vi "WriteSingleJoint.vi"(0 "Angle Name":T1(ring), 1 "node":string, 2 "Angle (degrees)":dbl, 3 "error in":errorcluster, 4 "Mode":T2=1 items=["Position"=1, "Velocity"=2, "Effort"=3]) -> (6 "error out":errorcluster)   [LabVIEW 2010]
uses:
  ROS/Code/SubVIs/_ROSDirection.ctl
  ROS/Code/Console/Servers/ServerSubs/TopicDef.ctl
  ROS/MessageBuilding/std_msgs/subs/i32Scalar.vi
  ROS/MessageBuilding/std_msgs/subs/float64Array.vi
  ROS/MessageBuilding/std_msgs/subs/stringArray.vi
  ROS/Code/SubVIs/JointMode.ctl
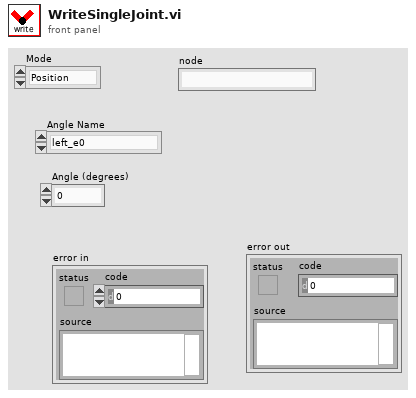
[diagram p1: front panel]
types:
  T1 = enum16{"left_e0", "left_e1", "left_s0", "left_s1", "left_w0", "left_w1", "left_w2", "right_e0", "right_e1", "right_s0", "right_s1", "right_w0", "right_w1", "right_w2"}
  T2 = typedef "JointMode.ctl" = u8
  T3 = typedef "TopicDef.ctl" = cluster{"Topic":string, "Type":string, "Action":T4, "Update (ms)":u16, "write queue":u16}
  T4 = typedef "_ROSDirection.ctl" = enum16{"Node", "Publisher", "Subscriber", "Service Client"}
  T5 = typedef "_ROSControl.ctl" = cluster{"topic port":u16, "Node":string, "topic":string, "type":string, "node port":u32, "error ":errorcluster, "Direction":T4, "APIs":string[], "Update (ms)":u16, "write queue":u16}
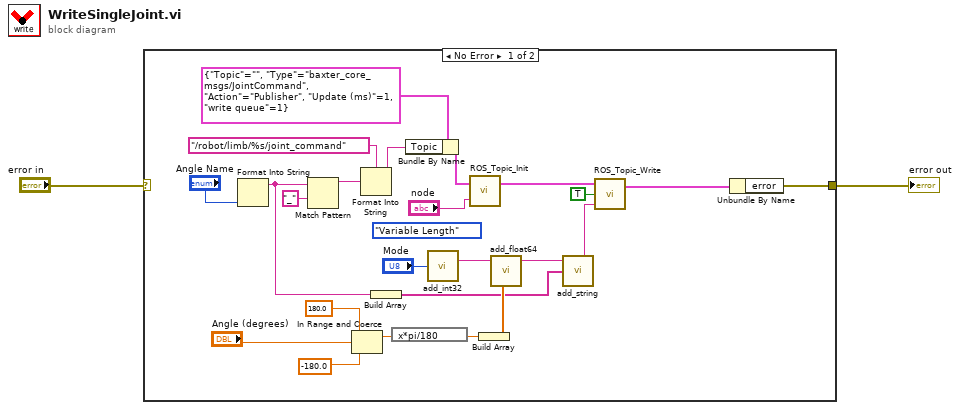
[diagram p0: block diagram]
diagram:
  n1 = case shown="No Error" "error in" {
    selector: "error in" -> [_ w27]
    tunnel: [w26 w27] -> w2
    frame No Error {
      (unwired) enum16{"Fixed Length", "Variable Length"}."Variable Length" ("Array Type")
      n2 = Format Into String("Angle Name") -> (resulting string=w6:string)  [unwired: 3 in, 1 out]
      n3 = Match Pattern(string=w6, regular expression="_") -> (before substring=w11:string)  [unwired: 1 in, 3 out]
      n4 = In Range and Coerce(upper limit=180.0 ("Elbow 0"), x="Angle (degrees)", lower limit=-180.0 ("Elbow 0")) -> (coerced(x)=w20:dbl)  [unwired: 1 out]
      n5 = Format Into String(format string="/robot/limb/%s/joint_command" ("Topic"), w11) -> (resulting string=w17:string)  [unwired: 2 in, 1 out]
      n6 = Build Array(w6) -> (w3:string[])
      n7 = expression code="x*pi/180"(w20) -> (w5:dbl)
      n8 = Bundle By Name(cluster=T3 {"Topic"="", "Type"="baxter_core_msgs/JointCommand", "Action"=enum."Publisher", "Update (ms)"=1, "write queue"=1} ("Definitions"), "Topic"=w17) -> (w15:T3)
      n9 = call-poly "add_int32.vi"("Numeric"="Mode") -> ("msg out"=w8:string)  [unwired: 4 in]
      n10 = call "ROS_Topic_Init.vi"("node"="node", "Definitions"=w15) -> ("ROS out"=w24:T5)  [unwired: 1 in]
      n11 = Build Array(w5) -> (w4:dbl[])
      n12 = call-poly "add_float64.vi"("Array"=w4, "msg in"=w8) -> ("msg out"=w9:string)  [unwired: 3 in]
      n13 = call-poly "add_string.vi"("Array"=w3, "msg in"=w9) -> ("msg out"=w7:string)  [unwired: 3 in]
      n14 = call "ROS_Topic_Write.vi"("Msg in"=w7, "Continuous?"=TRUE, "ROS in"=w24) -> ("ROS out"=w23:T5)  [unwired: 1 in]
      n15 = Unbundle By Name(w23) -> ("error"=w26:errorcluster)
    }
    frame Error {
    }
  }
  "error out" <- w2
